vi "ASC_thermal2.0.vi"() -> ()   [LabVIEW 2009]
uses:
  PID_globals.vi
  <vilib>/Utility/error.llb/DialogType.ctl
  <vilib>/Instr/_visa.llb/VISA Configure Serial Port (Instr).vi
  Time_globals.vi
  Instance           4 19Saved   Wetlow_v1.2 .vi
panel:
  in  "error in":errorcluster
  out "Datafile blob":string
  out "Field on/off":bool
  out "Soak Time (min)":u32=30
  out "SP-20 Time":dbl format="%#_4g"
  out "SP Time":dbl format="%#_4g"
  out "Field (uT)":dbl
  out "Set Point (*C)":u32
  out "Time from SP":dbl format="%#_4g"
  out "Elapsed Time":dbl format="%#_3g"
  out "fan end":u32
  out "load end":u32
  out "sample":u32
  out "Wetlow Chart":T1(graph)
  in  "stop":bool
  # "Temperature"
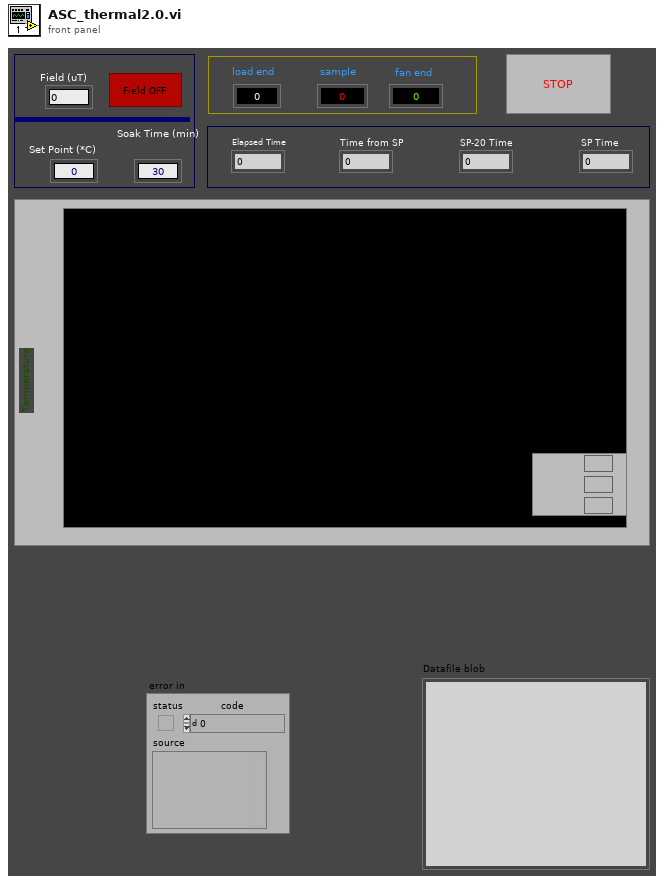
[diagram p1: front panel]
types:
  T1 = cluster{"Number":u32, "Number":u32, "Number":u32}
  T2 = cluster{"Number":u32, "Number":u32, "Number":u32}[]
  T3 = cluster{"Set Point (*C)":u32, "Field (uT)":dbl, "Soak Time (min)":u32, "Field on/off":bool, "Atmosphere":string, "Use DB":enum32{"DB Yes", "DB no"}, "User ID":string, "Batch / Boat ID":string, "User":string, "Note":string, "Field on (C)":dbl, "Field off (C)":dbl, "email address":string, "Control ramp":bool, "Ramp rate":dbl, "Contact Me":enum32{"No Selection", "E-mail", "Text"}, "Test e-mail":bool, "Cellular Provider":string}
  T4 = typedef "DialogType.ctl" = u16
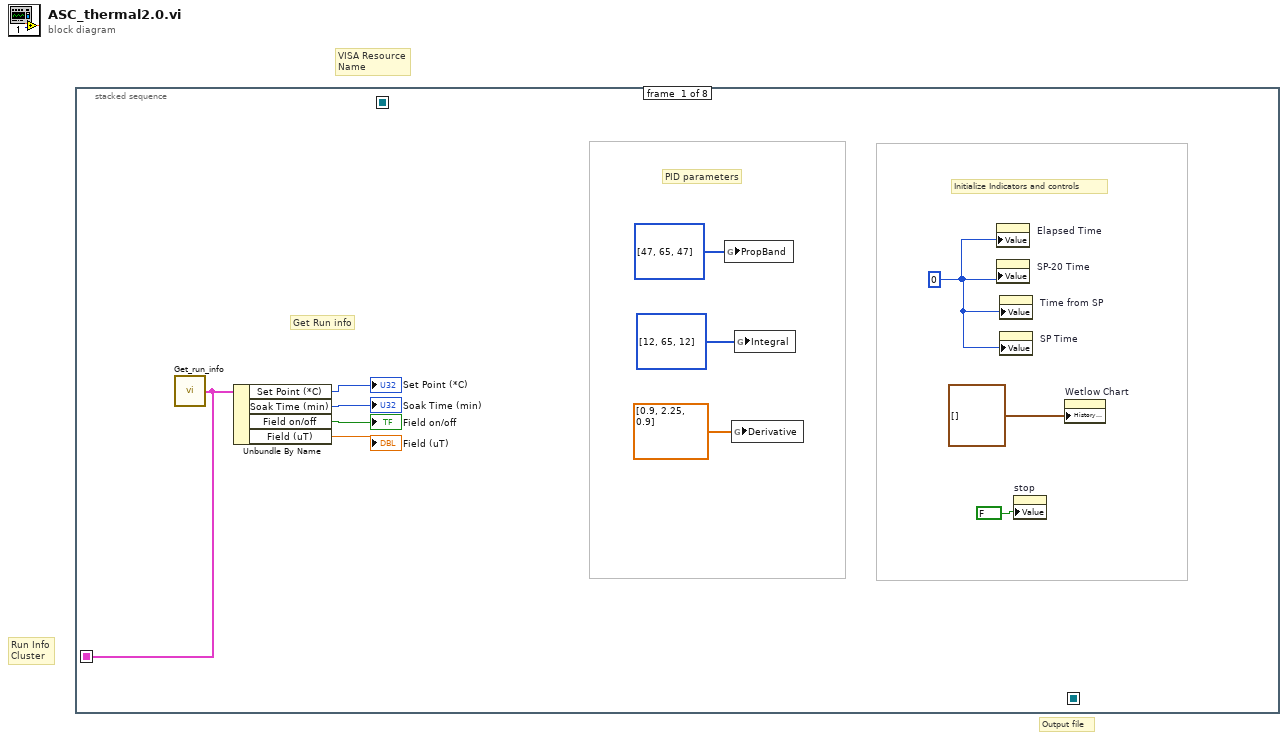
[diagram p0: block diagram]
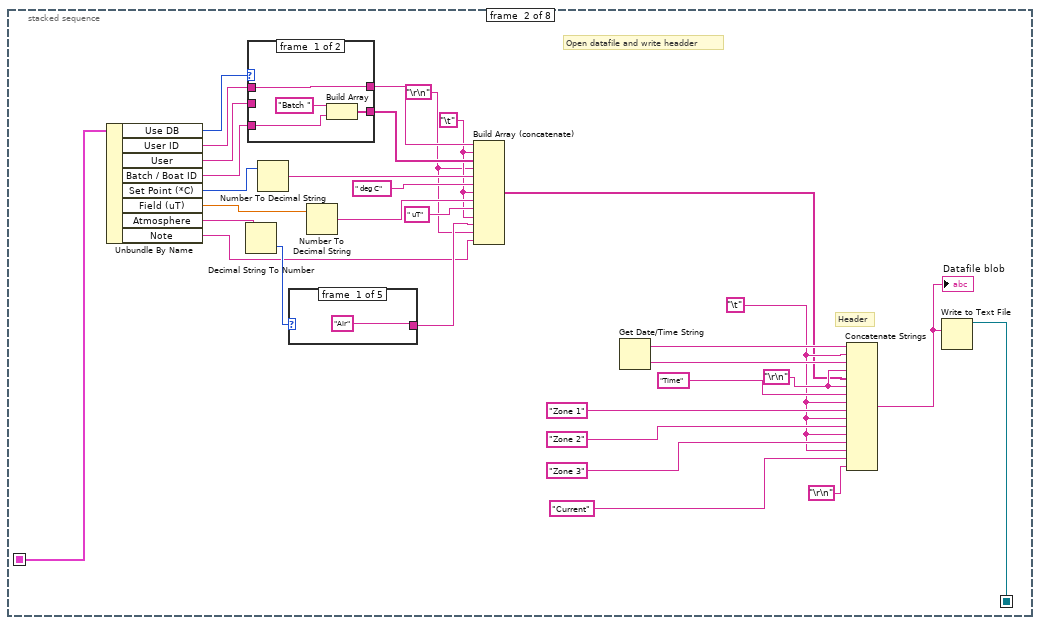
[diagram p2: hidden frame]
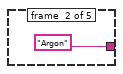
[diagram p3: hidden frame]
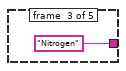
[diagram p4: hidden frame]
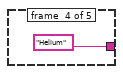
[diagram p5: hidden frame]
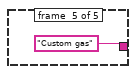
[diagram p6: hidden frame]
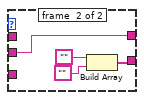
[diagram p7: hidden frame]
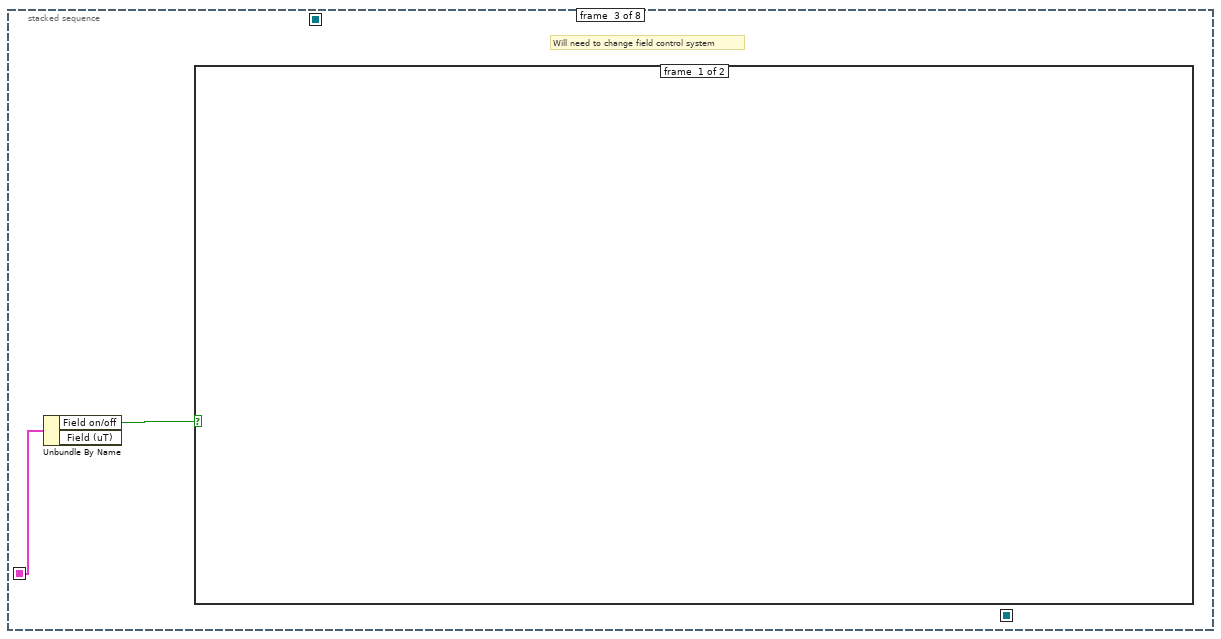
[diagram p8: hidden frame]
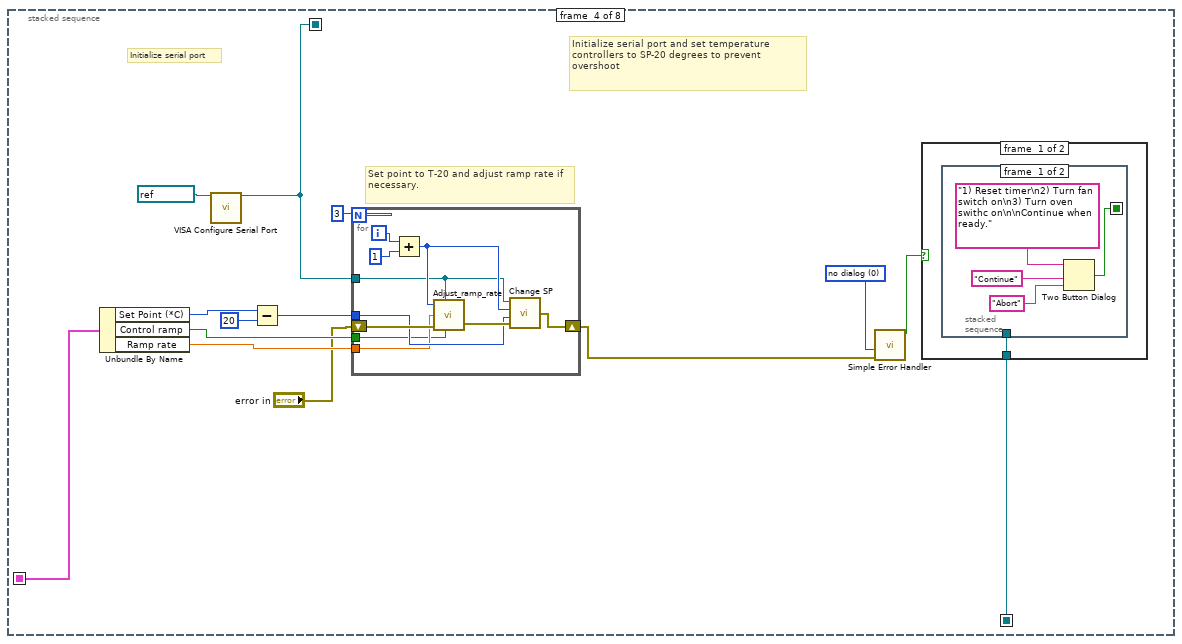
[diagram p10: hidden frame]
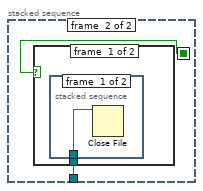
[diagram p11: hidden frame]
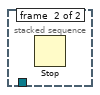
[diagram p12: hidden frame]
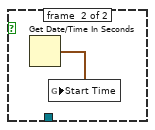
[diagram p13: hidden frame]
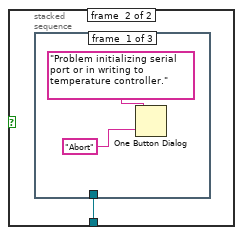
[diagram p14: hidden frame]
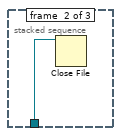
[diagram p15: hidden frame]
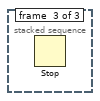
[diagram p16: hidden frame]
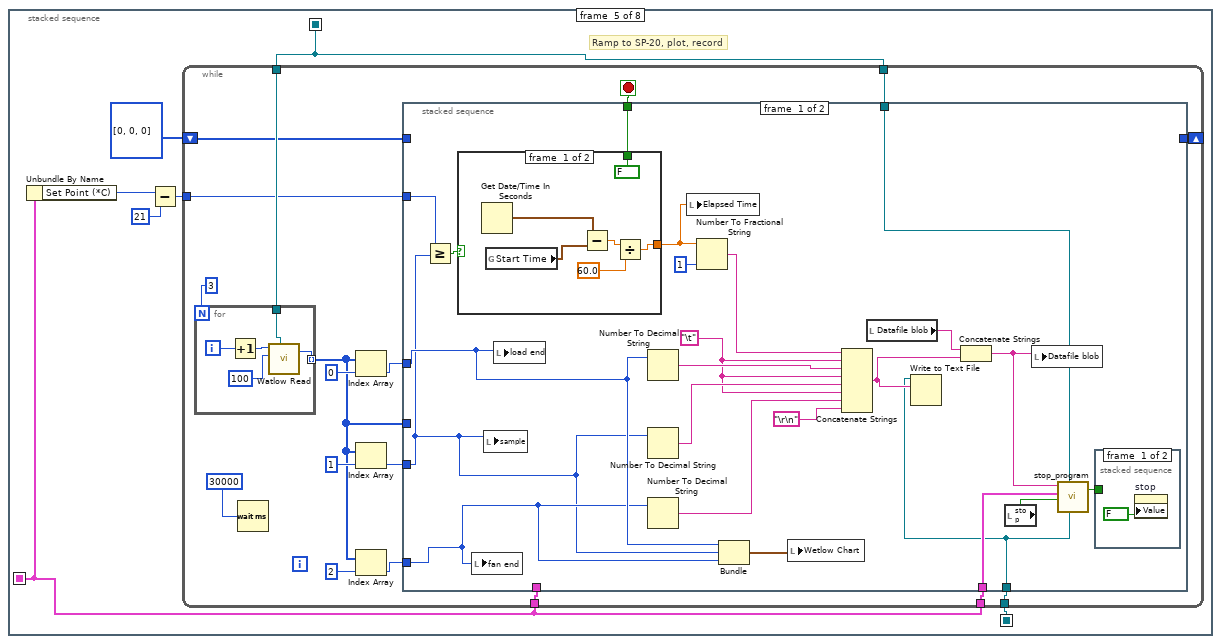
[diagram p17: hidden frame]
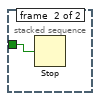
[diagram p18: hidden frame]
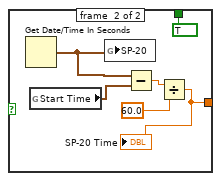
[diagram p19: hidden frame]
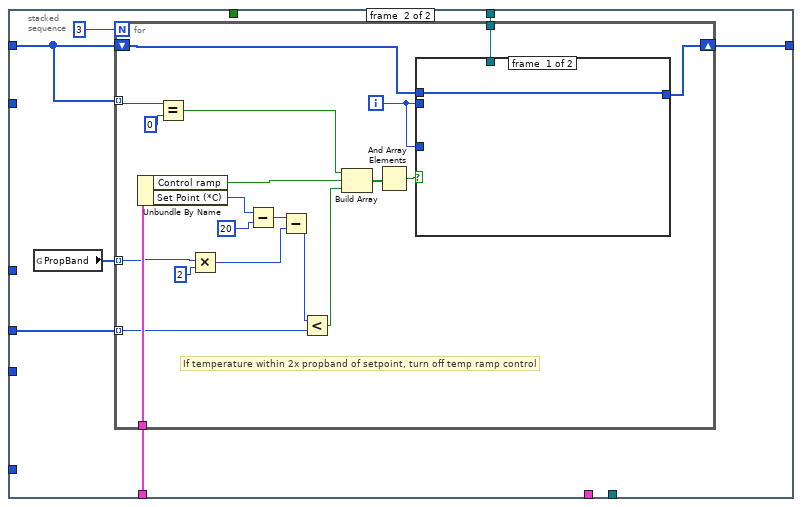
[diagram p20: hidden frame]
diagram:
  # "Run Info\nCluster"
  # "VISA Resource\nName"
  # "Output file"
  n1 = stacked-sequence {
    seq-local: [_ w36 _ _ _ _ _ _] -> [_ _ _ w67 w103 w203 w252 w333]
    seq-local: [_ _ _ w59 _ _ _ _] -> [_ _ _ _ w102 w201 w248 w331]
    seq-local: [w5 _ _ _ _ _ _ _] -> [_ w33 w58 w65 w98 w202 w249 w328]
    frame #0 {
      w6 = 0
      # "PID parameters"
      # "Initialize Indicators and controls"
      # "Get Run info"
      n2 = call "Get_run_info.vi"() -> ("Run Info Cluster Out"=w5:T3)  [unwired: 1 in]
      n3 = Unbundle By Name(w5) -> ("Set Point (*C)"=→"Set Point (*C)":u32, "Soak Time (min)"=→"Soak Time (min)":u32, "Field on/off"=→"Field on/off":bool, "Field (uT)"=→"Field (uT)":dbl)
      n4 = global write "PID_globals.vi" "PropBand"(i32[] [47, 65, 47]) -> ()
      n5 = global write "PID_globals.vi" "Derivative"(dbl[] [0.9, 2.25, 0.9]) -> ()
      n6 = global write "PID_globals.vi" "Integral"(i32[] [12, 65, 12]) -> ()
      n7 = property on="Elapsed Time" class="DigNum (strict)"("Value"=w6) -> ()  [unwired: 2 in, 2 out]
      n8 = property on="SP-20 Time" class="DigNum (strict)"("Value"=w6) -> ()  [unwired: 2 in, 2 out]
      n9 = property on="Time from SP" class="DigNum (strict)"("Value"=w6) -> ()  [unwired: 2 in, 2 out]
      n10 = property on="SP Time" class="DigNum (strict)"("Value"=w6) -> ()  [unwired: 2 in, 2 out]
      n11 = property on="stop" class="Bool (strict)"("Value"=FALSE ("stop")) -> ()  [unwired: 2 in, 2 out]
      n12 = property on="Wetlow Chart" class="WaveformChart (strict)"("History Data"=T2 []) -> ()  [unwired: 2 in, 2 out]
    }
    frame #1 {
      w16 = "\r\n" ("End of Line Constant")
      w20 = "\t" ("Tab Constant")
      w38 = "\r\n" ("End of Line Constant")
      w14 = "\t" ("Tab Constant")
      # "Open datafile and write headder"
      # "Header"
      n13 = Unbundle By Name(w33) -> ("Use DB"=w32:enum32{"DB Yes", "DB no"}, "User ID"=w30:string, "User"=w29:string, "Batch / Boat ID"=w28:string, "Set Point (*C)"=w26:u32, "Field (uT)"=w25:dbl, "Atmosphere"=w19:string, "Note"=w15:string)
      n14 = Decimal String To Number(string=w19) -> (number=w18:i32)  [unwired: 3 out]
      n15 = case shown="\"DB Yes\", Default" w32 {
        tunnel: w29 -> [_ w56]
        tunnel: [w52 w56] -> w31
        tunnel: w30 -> [w52 _]
        tunnel: w28 -> [w50 _]
        tunnel: [w49 w53] -> w27
        frame #0 {
          n16 = Build Array("Batch ", w50) -> (w49:string[])
        }
        frame #1 {
          n17 = Build Array("", "") -> (w53:string[])
        }
      }
      n18 = Number To Decimal String(number=w26) -> (decimal integer string=w24:string)  [unwired: 1 out]
      n19 = case shown="0, Default" w18 {
        tunnel: ["Air" "Argon" "Nitrogen" "Helium" "Custom gas"] -> w17
        frame #0 {
        }
        frame #1 {
        }
        frame #2 {
        }
        frame #3 {
        }
        frame #4 {
        }
      }
      n20 = Number To Decimal String(number=w25) -> (decimal integer string=w22:string)  [unwired: 1 out]
      n21 = Build Array (concatenate)(w31, w20, w27, w16, w24, " deg C", w20, w22, " uT", w20, w17, w16, w15) -> (w13:string[])
      n22 = Get Date/Time String() -> (date string=w40:string, time string=w39:string)  [unwired: 3 out]
      n23 = Concatenate Strings(w40, w14, w39, w38, w13, w38, "Time", w14, "Zone 1", w14, "Zone 2", w14, "Zone 3", w14, "Current", "\r\n") -> (w12:string)
      "Datafile blob" <- w12
      n24 = Write to Text File(text=w12) -> (refnum out=w36:refnum<file>)  [unwired: 1 in, 4 out]
    }
    frame #2 {
      # "Will need to change field control system"
      n25 = Unbundle By Name(w58) -> ("Field on/off"=w57:bool)  [unwired: 1 out]
      n26 = case shown="True" w57 {
        frame #0 {
        }
        frame #1 {
        }
      }
    }
    frame #3 {
      w69 = T4 0 items=["no dialog", "OK message", "continue or stop message", "OK message + warnings", "continue/stop + warnings"] ("type of dialog (OK msg:1)")
      # "Initialize serial port and set temperature controllers to SP-20 degrees to prevent overshoot"
      # "Initialize serial port"
      # "Set point to T-20 and adjust ramp rate if necessary."
      n27 = Unbundle By Name(w65) -> ("Set Point (*C)"=w66:u32, "Control ramp"=w64:bool, "Ramp rate"=w63:dbl)
      n28 = call-poly "VISA Configure Serial Port"("VISA resource name"=refnum<visa-resource-name> "COM3" ("VISA Resource Name")) -> ("VISA resource name out"=w59:refnum<visa-resource-name>)  [unwired: 5 in, 9 out]
      n29 = Subtract(x=w66, y=u32 20) -> (x-y=w70:u32)
      n30 = for {
        N: 3 ("Numeric") -> [_]
        shift-right: [w92] -> w62
        shift-left: "error in" -> [w94]
        tunnel: w70 -> [w90]
        tunnel: w59 -> [w87]
        tunnel: w64 -> [w88]
        tunnel: w63 -> [w89]
        i -> [w96]
        n31 = Add(x=w96, y=1) -> (x+y=w91:i32)
        n32 = call "Adjust_ramp_rate.vi"("Address"=w91, "VISA resource"=w87, "Ramp rate"=w89, "error in"=w94, "Control ramp"=w88) -> ("error out"=w93:errorcluster)  [unwired: 1 out]
        n33 = call "Change SP.vi"("error in"=w93, "Set Point"=w90, "Adress"=w91, "VISA resource name"=w87) -> ("error out"=w92:errorcluster)
      }
      n34 = call <vilib>:"Simple Error Handler.vi"("type of dialog (OK msg:1)"=w69, "error in (no error)"=w62) -> ("error?"=w68:bool)  [unwired: 7 out]
      n35 = case shown="False" w68 {
        tunnel: w67 -> [w73 w83]
        frame #0 {
          n36 = stacked-sequence {
            seq-local: [w74 _] -> [_ w79]
            tunnel: w73 -> [_ w78]
            frame #0 {
              n37 = Two Button Dialog(message="1) Reset timer\n2) Turn fan switch on\n3) Turn oven swithc on\n\nContinue when ready.", 1:"Abort", 2:"Continue") -> (T button?=w74:bool)
            }
            frame #1 {
              n38 = case shown="False" w79 {
                tunnel: w78 -> [w80 _]
                frame #0 {
                  n39 = stacked-sequence {
                    tunnel: w80 -> [w81 _]
                    frame #0 {
                      n40 = Close File(refnum=w81) -> ()  [unwired: 1 in, 2 out]
                    }
                    frame #1 {
                      n41 = Stop() -> ()  [unwired: 1 out]
                    }
                  }
                }
                frame #1 {
                  n42 = Get Date/Time In Seconds() -> (seconds since 1Jan1904=w82:timestamp)
                  n43 = global write "Time_globals.vi" "Start Time"(w82) -> ()
                }
              }
            }
          }
        }
        frame #1 {
          n44 = stacked-sequence {
            tunnel: w83 -> [_ w86 _]
            frame #0 {
              n45 = One Button Dialog(message="Problem initializing serial port or in writing to temperature controller.", button name ("OK")="Abort") -> ()  [unwired: 1 out]
            }
            frame #1 {
              n46 = Close File(refnum=w86) -> ()  [unwired: 1 in, 2 out]
            }
            frame #2 {
              n47 = Stop() -> ()  [unwired: 1 out]
            }
          }
        }
      }
    }
    frame #4 {
      # "Ramp to SP-20, plot, record"
      n48 = Unbundle By Name(w98) -> ("Set Point (*C)"=w101:u32)
      n49 = Subtract(x=w101, y=u32 21) -> (x-y=w99:u32)
      n50 = while {
        tunnel: w103 -> [w111]
        tunnel: w102 -> [w113]
        tunnel: w98 -> [w112]
        tunnel: w102 -> [w110]
        tunnel: w99 -> [w109]
        tunnel: w98 -> [w108]
        shift-right: [w104] -> _
        shift-left: i32[] [0, 0, 0] -> [w105]
        stop <- w106 stop-if-true
        n51 = for {
          N: 3 -> [_]
          tunnel: [w124] -> w107 mode=indexing
          tunnel: w113 -> [w123]
          i -> [w126]
          n52 = Increment(x=w126) -> (x+1=w125:i32)
          n53 = call "Watlow Read.vi"("Adress"=w125, "Register"=u8 100 ("ST-H"), "VISA resource name"=w123) -> ("Number"=w124:u32)  [unwired: 1 in, 2 out]
        }
        n54 = Wait (ms)(milliseconds to wait=u32 30000) -> ()  [unwired: 1 out]
        n55 = Index Array(array=w107, index=0) -> (element=w116:u32)
        n56 = Index Array(array=w107, index=1) -> (element=w114:u32)
        n57 = Index Array(array=w107, index=2) -> (element=w115:u32)
        n58 = stacked-sequence {
          tunnel: w116 -> [w143 _]
          tunnel: w115 -> [w142 _]
          tunnel: w114 -> [w141 _]
          tunnel: w112 -> [w131 _]
          tunnel: w111 -> [w130 _]
          tunnel: w110 -> [w129 w164]
          tunnel: w109 -> [w128 _]
          tunnel: w108 -> [_ w169]
          tunnel: w107 -> [_ w168]
          tunnel: [w127 _] -> w106
          tunnel: w105 -> [_ w166]
          tunnel: [_ w165] -> w104
          frame #0 {
            w146 = "\t"
            n59 = Greater Or Equal?(x=w141, y=w128) -> (x >= y?=w140:bool)
            n60 = case shown="True" w140 {
              tunnel: [w153 w159] -> w138
              tunnel: [FALSE TRUE] -> w127
              frame #0 {
                n61 = Get Date/Time In Seconds() -> (seconds since 1Jan1904=w154:timestamp)
                n62 = global read "Time_globals.vi" "Start Time"() -> (w155:timestamp)
                n63 = Subtract(x=w154, y=w155) -> (x-y=w156:dbl)
                n64 = Divide(x=w156, y=60.0) -> (x/y=w153:dbl)
              }
              frame #1 {
                n65 = Get Date/Time In Seconds() -> (seconds since 1Jan1904=w163:timestamp)
                n66 = global read "Time_globals.vi" "Start Time"() -> (w162:timestamp)
                n67 = global write "Time_globals.vi" "SP-20"(w163) -> ()
                n68 = Subtract(x=w163, y=w162) -> (x-y=w161:dbl)
                n69 = Divide(x=w161, y=60.0) -> (x/y=w159:dbl)
                "SP-20 Time" <- w159
              }
            }
            n70 = local write "fan end"(w142) -> ()
            n71 = local write "sample"(w141) -> ()
            n72 = local write "load end"(w143) -> ()
            n73 = Number To Decimal String(number=w143) -> (decimal integer string=w149:string)  [unwired: 1 out]
            n74 = Number To Decimal String(number=w141) -> (decimal integer string=w148:string)  [unwired: 1 out]
            n75 = Number To Decimal String(number=w142) -> (decimal integer string=w147:string)  [unwired: 1 out]
            n76 = local write "Elapsed Time"(w138) -> ()
            n77 = Number To Fractional String(number=w138, precision (6)=i16 1) -> (F-format string=w139:string)  [unwired: 2 out]
            n78 = Bundle("Number"=w143, "Number"=w141, "Number"=w142) -> (w144:T1)  [unwired: 1 out]
            n79 = local write "Wetlow Chart"(w144) -> ()
            n80 = Concatenate Strings(w139, w146, w149, w146, w148, w146, w147, "\r\n") -> (w133:string)
            n81 = local read "Datafile blob"() -> (w134:string)
            n82 = Write to Text File(file (use dialog)=w130, text=w133) -> ()  [unwired: 1 in, 4 out]
            n83 = Concatenate Strings(w134, w133) -> (w132:string)
            n84 = local read "stop"() -> (w136:bool)
            n85 = local write "Datafile blob"(w132) -> ()
            n86 = call "stop_program.vi"("filename"=w130, "VISA resource name"=w129, "stop"=w136, "Run Info Cluster In"=w131, "Datafile blob"=w132) -> ("Reset?"=w135:bool)  [unwired: 1 in, 1 out]
            n87 = stacked-sequence {
              tunnel: w135 -> [_ w151]
              frame #0 {
                n88 = property on="stop" class="Bool (strict)"("Value"=FALSE) -> ()  [unwired: 2 in, 2 out]
              }
              frame #1 {
                n89 = Stop(stop? (T)=w151) -> ()
              }
            }
          }
          frame #1 {
            n90 = global read "PID_globals.vi" "PropBand"() -> (w167:i32[])
            n91 = for {
              N: 3 -> [_]
              tunnel: w169 -> [w190]
              tunnel: w168 -> [w182] mode=indexing
              tunnel: w167 -> [w188] mode=indexing
              tunnel: w166 -> [w177] mode=indexing
              shift-right: [w173] -> w165
              shift-left: w166 -> [w174]
              tunnel: w164 -> [w172]
              i -> [w171]
              # "If temperature within 2x propband of setpoint, turn off temp ramp control"
              n92 = Unbundle By Name(w190) -> ("Control ramp"=w180:bool, "Set Point (*C)"=w187:u32)
              n93 = Equal?(x=w177, y=0) -> (x = y?=w176:bool)
              n94 = Multiply(x=w188, y=2) -> (x*y=w184:i32)
              n95 = Subtract(x=w187, y=20) -> (x-y=w185:u32)
              n96 = Subtract(x=w185, y=w184) -> (x-y=w183:u32)
              n97 = Less?(x=w183, y=w182) -> (x < y?=w179:bool)
              n98 = Build Array(w176, w180, w179) -> (w175:bool[])
              n99 = And Array Elements(Boolean array=w175) -> (logical AND=w181:bool)
              n100 = case shown="True" w181 {
                tunnel: w174 -> [w191 w199]
                tunnel: [w191 w197] -> w173
                tunnel: w171 -> [_ w200]
                tunnel: w172 -> [_ w196]
                tunnel: w171 -> [_ w195]
                frame #0 {
                }
                frame #1 {
                  n101 = Increment(x=w195) -> (x+1=w194:i32)
                  n102 = Replace Array Subset(array=w199, new element=1 ("new element/subarray"), index=w200) -> (w197:i32[])
                  n103 = call "Adjust_ramp_rate.vi"("Address"=w194, "VISA resource"=w196, "Control ramp"=FALSE) -> ("error out"=w192:errorcluster)  [unwired: 2 in, 1 out]
                  n104 = call <vilib>:"General Error Handler.vi"("error in (no error)"=w192) -> ()  [unwired: 10 in, 5 out]
                }
              }
            }
          }
        }
      }
    }
    frame #5 {
      # "Soak at SP-20 for 20 min"
      n105 = while {
        tunnel: w201 -> [w212]
        tunnel: w203 -> [w211]
        tunnel: w202 -> [w205]
        tunnel: w201 -> [w204]
        stop <- w219 stop-if-true
        w231 = "\t"
        n106 = for {
          N: 3 -> [_]
          tunnel: [w245] -> w234 mode=indexing
          tunnel: w212 -> [w244]
          i -> [w247]
          n107 = Increment(x=w247) -> (x+1=w246:i32)
          n108 = call "Watlow Read.vi"("Adress"=w246, "Register"=u8 100 ("ST-H"), "VISA resource name"=w244) -> ("Number"=w245:u32)  [unwired: 1 in, 2 out]
        }
        n109 = Wait (ms)(milliseconds to wait=u32 30000) -> ()  [unwired: 1 out]
        n110 = global read "Time_globals.vi" "SP-20"() -> (w224:timestamp)
        n111 = Get Date/Time In Seconds() -> (seconds since 1Jan1904=w216:timestamp)
        n112 = Subtract(x=w216, y=w224) -> (x-y=w223:dbl)
        n113 = Divide(x=w223, y=60.0) -> (x/y=w221:dbl)
        n114 = Index Array(array=w234, index=0) -> (element=w229:u32)
        n115 = Index Array(array=w234, index=1) -> (element=w227:u32)
        n116 = Index Array(array=w234, index=2) -> (element=w228:u32)
        n117 = Greater Or Equal?(x=w221, y=20.0) -> (x >= y?=w219:bool)
        n118 = global read "Time_globals.vi" "Start Time"() -> (w215:timestamp)
        n119 = local write "fan end"(w228) -> ()
        n120 = local write "sample"(w227) -> ()
        n121 = local write "load end"(w229) -> ()
        n122 = Subtract(x=w216, y=w215) -> (x-y=w217:dbl)
        n123 = Divide(x=w217, y=60.0) -> (x/y=w213:dbl)
        n124 = Number To Decimal String(number=w229) -> (decimal integer string=w240:string)  [unwired: 1 out]
        n125 = Number To Decimal String(number=w227) -> (decimal integer string=w233:string)  [unwired: 1 out]
        n126 = Number To Decimal String(number=w228) -> (decimal integer string=w232:string)  [unwired: 1 out]
        n127 = Number To Fractional String(number=w213, precision (6)=i16 1) -> (F-format string=w226:string)  [unwired: 2 out]
        n128 = local write "Elapsed Time"(w213) -> ()
        n129 = Bundle("Number"=w229, "Number"=w227, "Number"=w228) -> (w214:T1)  [unwired: 1 out]
        n130 = local write "Wetlow Chart"(w214) -> ()
        n131 = Concatenate Strings(w226, w231, w240, w231, w233, w231, w232, "\r\n") -> (w207:string)
        n132 = local read "Datafile blob"() -> (w208:string)
        n133 = Write to Text File(file (use dialog)=w211, text=w207) -> ()  [unwired: 1 in, 4 out]
        n134 = Concatenate Strings(w208, w207) -> (w206:string)
        n135 = local read "stop"() -> (w210:bool)
        n136 = local write "Datafile blob"(w206) -> ()
        n137 = call "stop_program.vi"("filename"=w211, "VISA resource name"=w204, "stop"=w210, "Run Info Cluster In"=w205, "Datafile blob"=w206) -> ("Reset?"=w209:bool)  [unwired: 1 in, 1 out]
        n138 = stacked-sequence {
          tunnel: w209 -> [_ w242]
          frame #0 {
            n139 = property on="stop" class="Bool (strict)"("Value"=FALSE) -> ()  [unwired: 2 in, 2 out]
          }
          frame #1 {
            n140 = Stop(stop? (T)=w242) -> ()
          }
        }
      }
    }
    frame #6 {
      n141 = Unbundle By Name(w249) -> ("Set Point (*C)"=w251:u32, "Soak Time (min)"=w250:u32)
      n142 = for {
        N: 20 -> [_]
        tunnel: w252 -> [w255]
        tunnel: w248 -> [w262]
        tunnel: w248 -> [w261]
        tunnel: w251 -> [w259]
        tunnel: w250 -> [w258]
        tunnel: w249 -> [w256]
        tunnel: w248 -> [w254]
        i -> [w265]
        n143 = Add(x=w265, y=1) -> (x+y=w269:i32)
        n144 = Subtract(x=20, y=w269) -> (x-y=w267:i32)
        n145 = flat-sequence {
          tunnel: w266 -> [w273]
          tunnel: w262 -> [w272]
          tunnel: w255 -> [w283]
          tunnel: [w284] -> w263
          tunnel: w261 -> [w285]
          tunnel: [w280] -> w257
          tunnel: w260 -> [w319]
          tunnel: w263 -> [w318]
          tunnel: w258 -> [w317]
          tunnel: w257 -> [w314]
          tunnel: w256 -> [w313]
          tunnel: w255 -> [w312]
          tunnel: w254 -> [w311]
          frame #0 {
            n146 = for {
              N: 3 -> [_]
              tunnel: w273 -> [w276]
              tunnel: w272 -> [w275]
              i -> [w279]
              n147 = Add(x=w279, y=1) -> (x+y=w277:i32)
              n148 = call "Change SP.vi"("Set Point"=w276, "Adress"=w277, "VISA resource name"=w275) -> ()  [unwired: 1 in, 1 out]
            }
            n149 = Wait (ms)(milliseconds to wait=u32 30000) -> ()  [unwired: 1 out]
          }
          frame #1 {
            w301 = "\t"
            n150 = for {
              N: 3 -> [_]
              tunnel: [w308] -> w298 mode=indexing
              tunnel: w285 -> [w307]
              i -> [w310]
              n151 = Increment(x=w310) -> (x+1=w309:i32)
              n152 = call "Watlow Read.vi"("Adress"=w309, "Register"=u8 100 ("ST-H"), "VISA resource name"=w307) -> ("Number"=w308:u32)  [unwired: 1 in, 2 out]
            }
            n153 = Index Array(array=w298, index=0) -> (element=w303:u32)
            n154 = Index Array(array=w298, index=1) -> (element=w305:u32)
            n155 = Index Array(array=w298, index=2) -> (element=w304:u32)
            n156 = local write "fan end"(w304) -> ()
            n157 = global read "Time_globals.vi" "Start Time"() -> (w291:timestamp)
            n158 = local write "sample"(w305) -> ()
            n159 = local write "load end"(w303) -> ()
            n160 = Get Date/Time In Seconds() -> (seconds since 1Jan1904=w292:timestamp)
            n161 = Subtract(x=w292, y=w291) -> (x-y=w290:dbl)
            n162 = Number To Decimal String(number=w303) -> (decimal integer string=w293:string)  [unwired: 1 out]
            n163 = Number To Decimal String(number=w305) -> (decimal integer string=w299:string)  [unwired: 1 out]
            n164 = Number To Decimal String(number=w304) -> (decimal integer string=w300:string)  [unwired: 1 out]
            n165 = Divide(x=w290, y=60.0) -> (x/y=w284:dbl)
            n166 = local write "Elapsed Time"(w284) -> ()
            n167 = Bundle("Number"=w303, "Number"=w305, "Number"=w304) -> (w288:T1)  [unwired: 1 out]
            n168 = local read "Datafile blob"() -> (w282:string)
            n169 = Number To Fractional String(number=w284, precision (6)=i16 1) -> (F-format string=w286:string)  [unwired: 2 out]
            n170 = local write "Wetlow Chart"(w288) -> ()
            n171 = Concatenate Strings(w286, w301, w293, w301, w299, w301, w300, "\r\n") -> (w281:string)
            n172 = Concatenate Strings(w282, w281) -> (w280:string)
            n173 = local write "Datafile blob"(w280) -> ()
            n174 = Write to Text File(file (use dialog)=w283, text=w281) -> ()  [unwired: 1 in, 4 out]
          }
          frame #2 {
            n175 = local read "stop"() -> (w316:bool)
            n176 = case shown="True" w319 {
              selector: w319 -> [_ w322]
              tunnel: w318 -> [_ w324]
              tunnel: w317 -> [_ w323]
              frame #0 {
              }
              frame #1 {
                n177 = Multiply(x=w323, y=u32 60) -> (x*y=w325:u32)
                n178 = call "Elapsed Time"("Time Target (s)"=w325, "Reset"=w322) -> ()  [unwired: 3 in, 15 out]
                "SP Time" <- w324
              }
            }
            n179 = call "stop_program.vi"("filename"=w312, "VISA resource name"=w311, "stop"=w316, "Run Info Cluster In"=w313, "Datafile blob"=w314) -> ("Reset?"=w315:bool)  [unwired: 1 in, 1 out]
            n180 = stacked-sequence {
              tunnel: w315 -> [_ w321]
              frame #0 {
                n181 = property on="stop" class="Bool (strict)"("Value"=FALSE) -> ()  [unwired: 2 in, 2 out]
              }
              frame #1 {
                n182 = Stop(stop? (T)=w321) -> ()
              }
            }
          }
        }
        n183 = Subtract(x=w259, y=w267) -> (x-y=w266:u32)
        n184 = Equal?(x=w265, y=19) -> (x = y?=w260:bool)
      }
    }
    frame #7 {
      n185 = Unbundle By Name(w328) -> ("Soak Time (min)"=w330:u32, "Contact Me"=w329:enum32{"No Selection", "E-mail", "Text"})
      n186 = case shown="\"E-mail\"" w329 {
        tunnel: w328 -> [_ w336 w338]
        tunnel: ["" w335 w337] -> w327
        frame #0 {
        }
        frame #1 {
          n187 = Unbundle By Name(w336) -> ("email address"=w335:string)
        }
        frame #2 {
          n188 = Unbundle By Name(w338) -> ("Cellular Provider"=w340:string, "email address"=w339:string)
          n189 = Concatenate Strings(w340, w339) -> (w337:string)
        }
      }
      n190 = while {
        tunnel: w333 -> [w371]
        shift-right: [w356] -> _
        shift-left: 0 -> [w355]
        tunnel: w331 -> [w354]
        tunnel: w328 -> [w347]
        tunnel: w329 -> [w341]
        tunnel: w327 -> [w348]
        tunnel: w331 -> [w346]
        tunnel: w330 -> [w344]
        stop <- w345 stop-if-true
        w376 = "\t"
        n191 = Multiply(x=u32 60, y=w344) -> (x*y=w342:u32)
        n192 = for {
          N: 3 -> [_]
          tunnel: [w403] -> w380 mode=indexing
          tunnel: w354 -> [w402]
          i -> [w405]
          n193 = Increment(x=w405) -> (x+1=w404:i32)
          n194 = call "Watlow Read.vi"("Adress"=w404, "Register"=u8 100 ("ST-H"), "VISA resource name"=w402) -> ("Number"=w403:u32)  [unwired: 1 in, 2 out]
        }
        n195 = Wait (ms)(milliseconds to wait=u32 30000) -> ()  [unwired: 1 out]
        n196 = call "Elapsed Time2"("Time Target (s)"=w342) -> ("Elapsed Time (s)"=w366:dbl, "Time has Elapsed"=w363:bool)  [unwired: 4 in, 13 out]
        n197 = Index Array(array=w380, index=0) -> (element=w375:u32)
        "load end" <- w375
        n198 = Index Array(array=w380, index=1) -> (element=w372:u32)
        "sample" <- w372
        n199 = Index Array(array=w380, index=2) -> (element=w374:u32)
        "fan end" <- w374
        n200 = Divide(x=w366, y=60.0) -> (x/y=→"Time from SP":dbl)
        n201 = case shown="True" w363 {
          tunnel: [FALSE w396] -> w358
          tunnel: w341 -> [_ w397]
          frame #0 {
          }
          frame #1 {
            n202 = call <vilib>:"Beep.vi"() -> ()  [unwired: 3 in, 9 out]
            n203 = case shown="\"No Selection\", Default" w397 {
              tunnel: [FALSE TRUE TRUE] -> w396
              frame #0 {
              }
              frame #1 {
              }
              frame #2 {
              }
            }
          }
        }
        n204 = Equal To 0?(x=w355) -> (x = 0?=w359:bool)
        n205 = And(x=w359, y=w358) -> (x .and. y?=w357:bool)
        n206 = global read "Time_globals.vi" "Start Time"() -> (w368:timestamp)
        n207 = Number To Decimal String(number=w375) -> (decimal integer string=w386:string)  [unwired: 1 out]
        n208 = Number To Decimal String(number=w372) -> (decimal integer string=w379:string)  [unwired: 1 out]
        n209 = Number To Decimal String(number=w374) -> (decimal integer string=w378:string)  [unwired: 1 out]
        n210 = case shown="True" w357 {
          tunnel: [w388 1] -> w356
          tunnel: w355 -> [w388 _]
          tunnel: w348 -> [_ w393]
          frame #0 {
          }
          frame #1 {
            n211 = call "GmailLV80.vi"("Subject"="Time's up!  Your samples are cooked.", "Recipient's Email Address"=w393, "Sender's Email Address (eg: LabVIEW@gmail.com)"="jbowles.irm@gmail.com", "GMAIL Account Password"="1%milkss", "GMAIL Account User ID"="jbowles.irm") -> ()  [unwired: 3 in, 4 out]
          }
        }
        n212 = Get Date/Time In Seconds() -> (seconds since 1Jan1904=w367:timestamp)
        n213 = Bundle("Number"=w375, "Number"=w372, "Number"=w374) -> (→"Wetlow Chart":T1)  [unwired: 1 out]
        n214 = Subtract(x=w367, y=w368) -> (x-y=w369:dbl)
        n215 = Divide(x=w369, y=60.0) -> (x/y=w362:dbl)
        "Elapsed Time" <- w362
        n216 = Number To Fractional String(number=w362, precision (6)=i16 1) -> (F-format string=w360:string)  [unwired: 2 out]
        n217 = Concatenate Strings(w360, w376, w386, w376, w379, w376, w378, "\r\n") -> (w350:string)
        n218 = local read "Datafile blob"() -> (w351:string)
        n219 = Write to Text File(file (use dialog)=w371, text=w350) -> (refnum out=w353:refnum<file>)  [unwired: 1 in, 3 out]
        n220 = Concatenate Strings(w351, w350) -> (w349:string)
        n221 = local write "Datafile blob"(w349) -> ()
        n222 = call "stop_program.vi"("filename"=w353, "VISA resource name"=w346, "stop"="stop", "Run Info Cluster In"=w347, "Datafile blob"=w349) -> ("Reset?"=w345:bool)  [unwired: 1 in, 1 out]
        n223 = case shown="True" w345 {
          frame #0 {
          }
          frame #1 {
            n224 = property on="stop" class="Bool (strict)"("Value"=FALSE) -> ()  [unwired: 2 in, 2 out]
          }
        }
      }
    }
  }
